vi "Two U8s to U16.vi"(1 "Index of first byte":i32, 2 "Byte array":u8[](array[numeric])) -> (0 "Output word":u16)   [LabVIEW 2016]
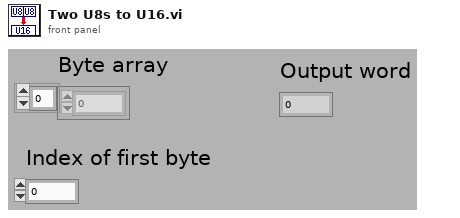
[diagram p1: front panel]
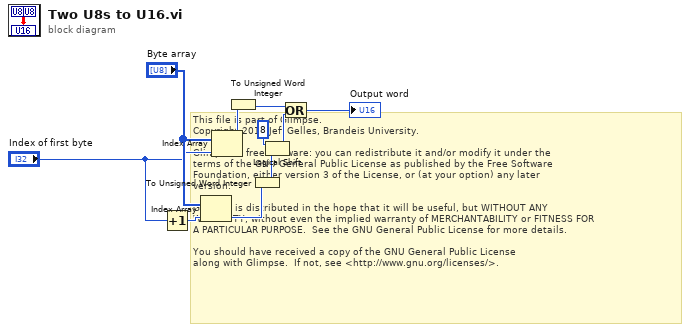
[diagram p0: block diagram]
diagram:
  # "This file is part of Glimpse. \nCopyright 2014 Jeff Gelles, Brandeis University.    \n\nGlimpse is free software: you can redistribute it and/or modify it under the \nterms of the GNU General Public License as published by the Free Software \nFoundation, either version 3 of the License, or (at your option) any later \nversion.\n\nGlimpse is distributed in the hope that it will be useful, but WITHOUT ANY \nWARRANTY; without even the implied warranty of MERCHANTABILITY or FITNESS FOR \nA PARTICULAR PURPOSE.  See the GNU General Public License for more details.\n\nYou should have received a copy of the GNU General Public License\nalong with Glimpse.  If not, see <http://www.gnu.org/licenses/>."
  n1 = Increment(x="Index of first byte") -> (x+1=w2:i32)
  n2 = Index Array(array="Byte array", index=w2) -> (element=w4:u8)
  n3 = Index Array(array="Byte array", index="Index of first byte") -> (element=w9:u8)
  n4 = To Unsigned Word Integer(number=w9) -> (unsigned 16bit integer=w8:u16)
  n5 = To Unsigned Word Integer(number=w4) -> (unsigned 16bit integer=w6:u16)
  n6 = Logical Shift(y=8, x=w6) -> (x << y=w5:u16)
  n7 = Or(x=w8, y=w5) -> (x .or. y?=→"Output word":u16)
